vi "SEA_LOWER_LEVEL_CONTROL.vi"() -> ()   [LabVIEW 2019]
uses:
  <vilib>/rvi/Emulation/niFpgaGetClockAttributes.vi
  <vilib>/rvi/Emulation/niFpgaSctlEmulationGetInTimedLoop.vi
  <vilib>/rvi/Emulation/niFpgaEmulationReportErrorSimple.vi
  <vilib>/rvi/eio/common/nirviEmuTemplateMethod_errors.vi
  <vilib>/rvi/Emulation/niFpgaCriticalErrorInLSC.vi
  <vilib>/eio/EIONode/EIONode.xnode
  <vilib>/rvi/Arithmetic/AddSubMult/XNode/nirviSatArithmetic.xnode
panel:
  in  "Position Reset joint side":bool
  out "Position (Counts) joint side":i16
  out "Acceleration (Counts/Interval) joint side":i32
  out "Velocity (Counts/Interval) joint side":i32
  out "Loop time (position) joint side":u32
  out "Position(Radians) joint side":sgl(graph)
  in  "Position Reset":bool
  out "Position (Counts) motor side":i16
  out "Acceleration (Counts/Interval) motor side":i32
  out "Velocity (Counts/Interval) motor side":i32
  out "Loop time (position) 1 motor side":u32
  out "Position(Radians) motor side":sgl(graph)
  in  "KpGain":sgl
  in  "Tracking zero offset":sgl
  in  "reference":sgl
  out "motor direction":bool
  out "control_ip":sgl
  out "Filtered Current(M2)":sgl(graph)
  in  "Current Offset":sgl=2.4882812 format="%#_13g"
  out "Current Control Loop rate":i32
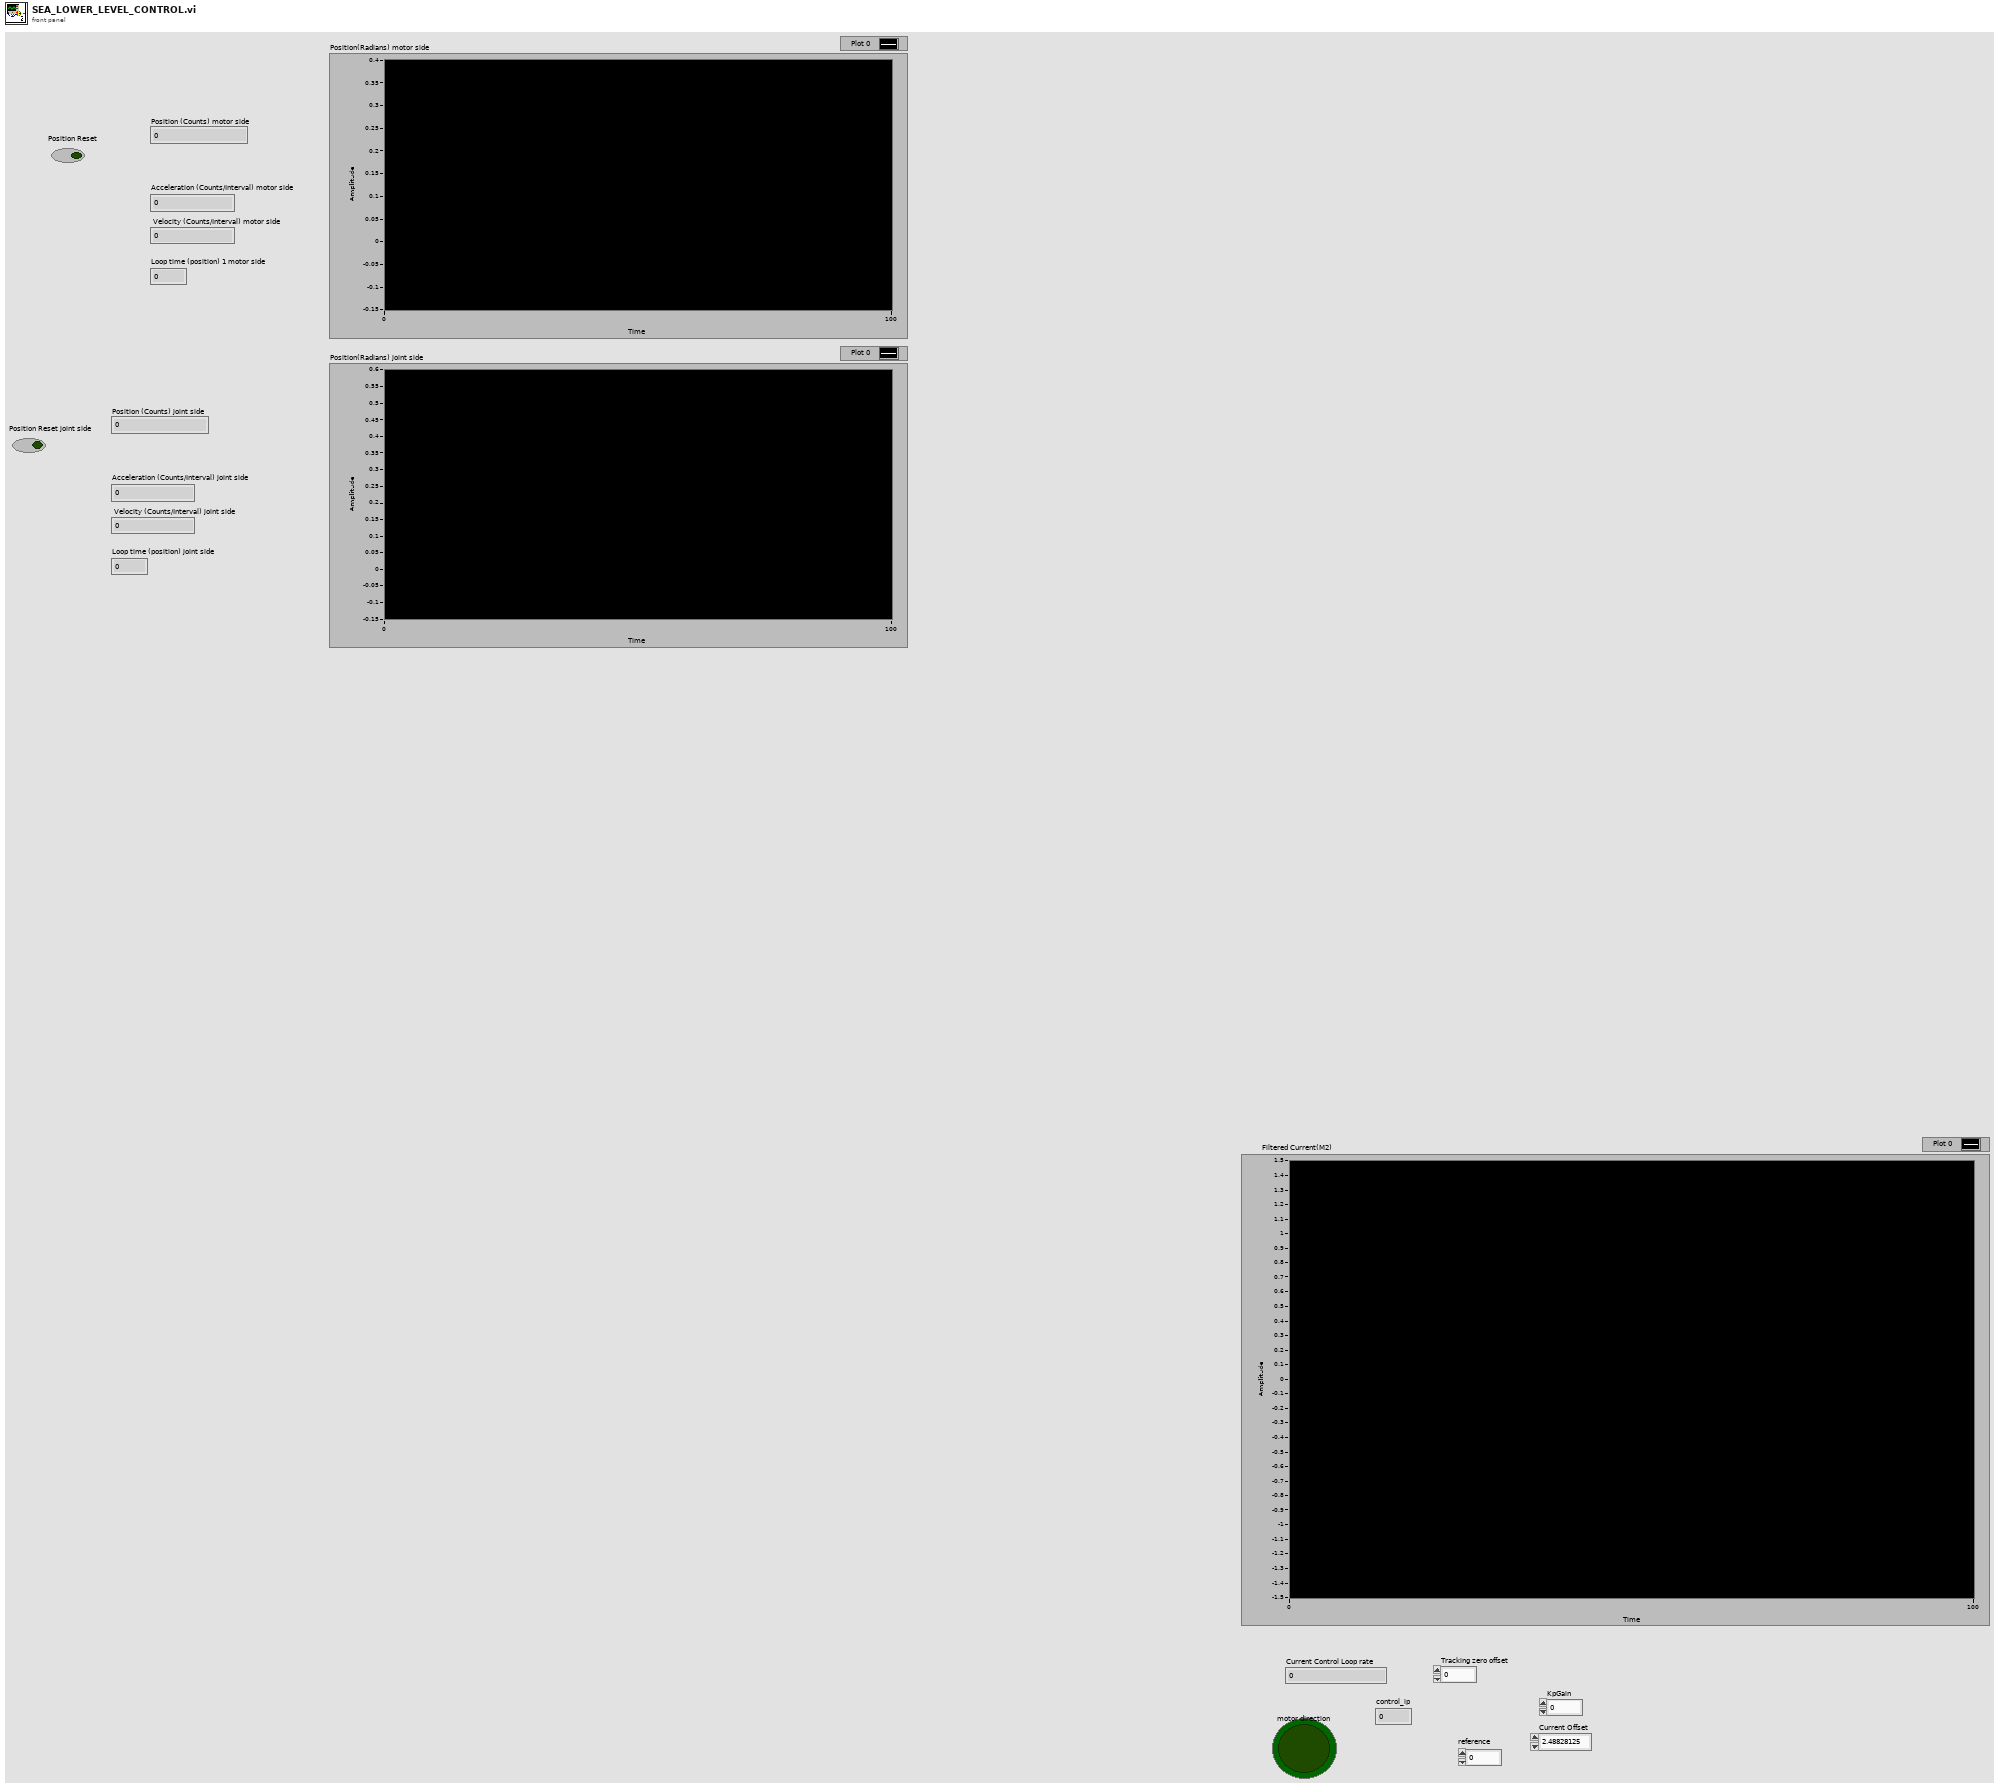
[diagram p1: front panel]
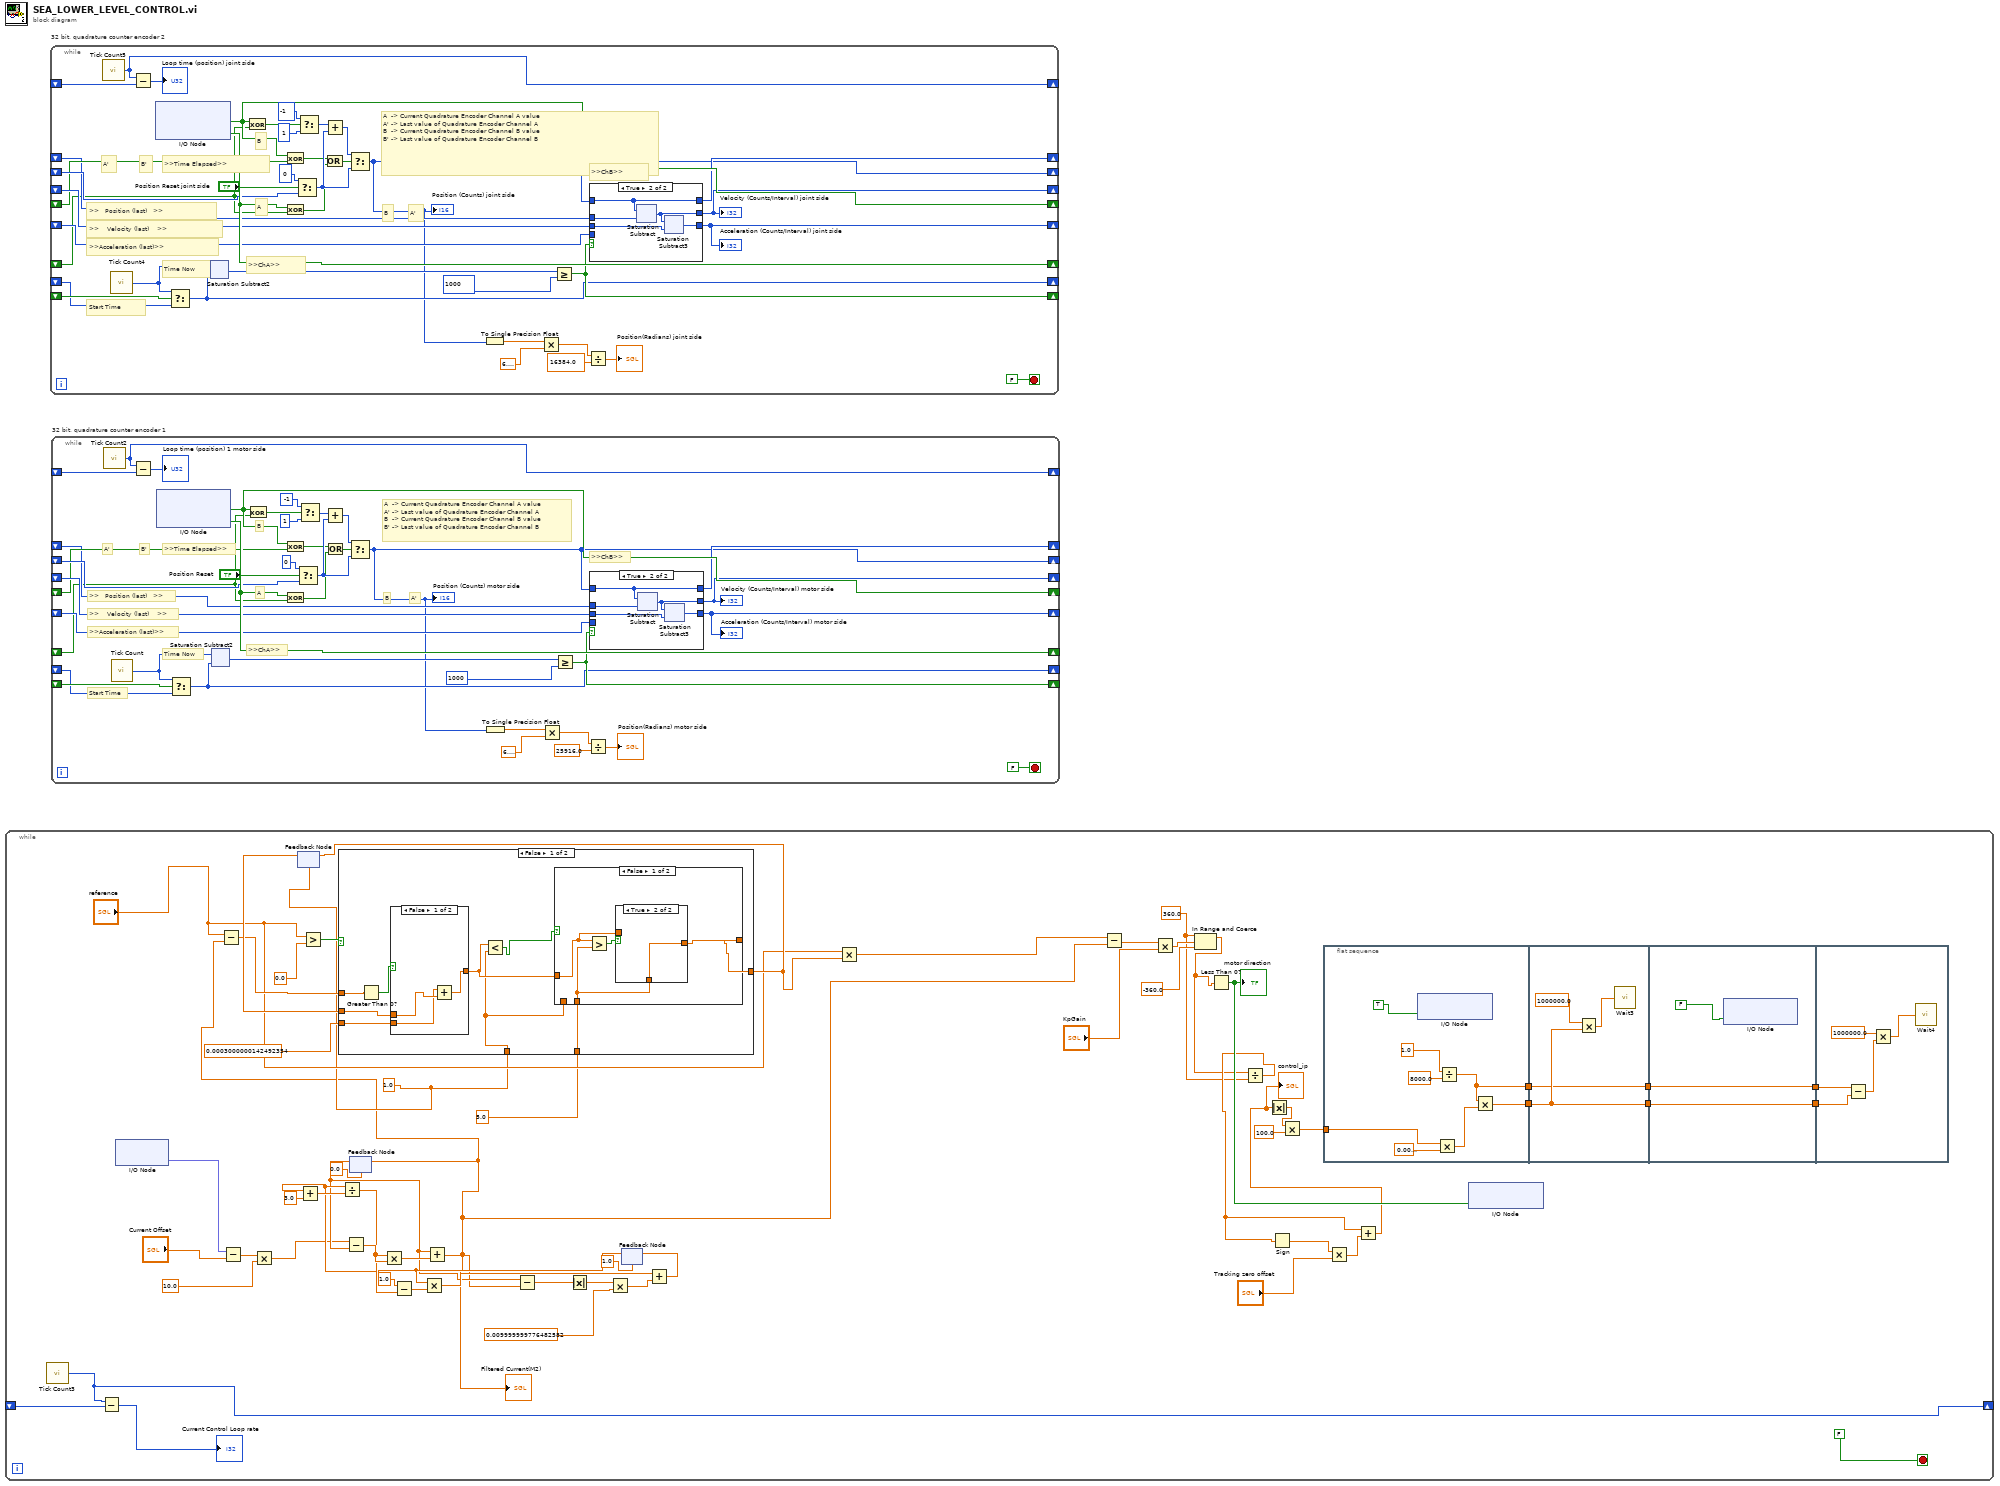
[diagram p0: block diagram]
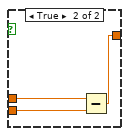
[diagram p4: hidden frame]
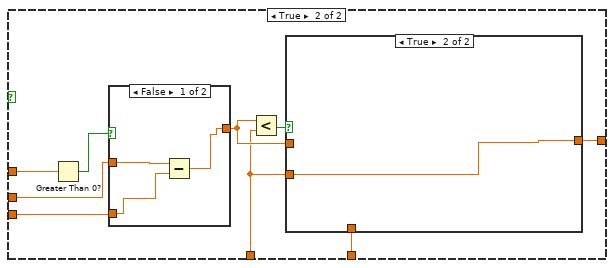
[diagram p7: hidden frame]
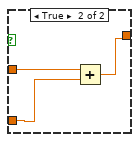
[diagram p8: hidden frame]
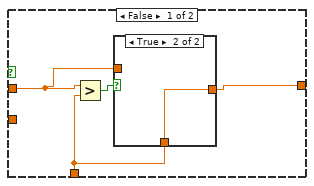
[diagram p9: hidden frame]
diagram:
  n1 = while {
    shift-right: [w22] -> _
    shift-left: _ -> [w23]
    stop <- FALSE stop-if-true
    w1 = sgl 360.0 ("upper limit")
    w11 = sgl 1.0
    n2 = call "Tick Count3"() -> ("Tick Count(uSec)"=w22:u32)
    n3 = Subtract(x=w22, y=w23) -> (x-y=→"Current Control Loop rate":u32)
    n4 = xnode "I/O Node"() -> ("AI9"=w24:fxp<+/-,24,5>)  [unwired: 1 in, 1 out]
    n5 = Subtract(x=w24, y="Current Offset") -> (x-y=w25:sgl)
    n6 = Multiply(x=w25, y=sgl 10.0) -> (x*y=w26:sgl)
    n7 = feedback #1(w11) -> (w56:sgl)
    n8 = Greater?(x="reference", y=sgl 0.0) -> (0:w57:bool)
    n9 = feedback #2(sgl 0.0) -> (w34:sgl)
    n10 = Subtract(x=w26, y=w34) -> (x-y=w42:sgl)
    n11 = feedback #3(sgl 1.0) -> (w35:sgl)
    n12 = Add(x=w35, y=sgl 3.0) -> (x+y=w44:sgl)
    n13 = Divide(x=w35, y=w44) -> (x/y=w41:sgl)
    n14 = Multiply(x=w41, y=w42) -> (x*y=w43:sgl)
    n15 = Subtract(x=sgl 1.0, y=w41) -> (x-y=w40:sgl)
    n16 = Multiply(x=w35, y=w40) -> (x*y=w39:sgl)
    n17 = Add(x=w34, y=w43) -> (x+y=w7:sgl)
    "Filtered Current(M2)" <- w7
    n18 = Subtract(x="reference", y=w7) -> (x-y=w20:sgl)
    n19 = case shown="False" w57 {
      tunnel: w20 -> [w86 w108]
      tunnel: w56 -> [w85 w106]
      tunnel: [w87 w109] -> w55
      tunnel: sgl 5.0 -> [w80 w103]
      tunnel: w11 -> [w81 w102]
      tunnel: sgl 0.0003 -> [w79 w101]
      frame False {
        n20 = Greater Than 0?(x=w86) -> (x > 0?=w84:bool)
        n21 = case shown="False" w84 {
          tunnel: w85 -> [w90 w93]
          tunnel: [w89 w92] -> w82
          tunnel: w79 -> [w88 w91]
          frame False {
            n22 = Add(x=w88, y=w90) -> (x+y=w89:sgl)
          }
          frame True {
            n23 = Subtract(x=w93, y=w91) -> (x-y=w92:sgl)
          }
        }
        n24 = Less?(x=w82, y=w81) -> (x < y?=w83:bool)
        n25 = case shown="False" w83 {
          tunnel: [w96 w100] -> w87
          tunnel: w82 -> [w95 _]
          tunnel: w81 -> [_ w100]
          tunnel: w80 -> [w94 _]
          frame False {
            n26 = Greater?(x=w95, y=w94) -> (0:w97:bool)
            n27 = case shown="True" w97 {
              tunnel: [w98 w99] -> w96
              tunnel: w95 -> [w98 _]
              tunnel: w94 -> [_ w99]
              frame False {
              }
              frame True {
              }
            }
          }
          frame True {
          }
        }
      }
      frame True {
        n28 = Greater Than 0?(x=w108) -> (x > 0?=w107:bool)
        n29 = case shown="False" w107 {
          tunnel: w106 -> [w112 w115]
          tunnel: [w111 w114] -> w104
          tunnel: w101 -> [w110 w113]
          frame False {
            n30 = Subtract(x=w112, y=w110) -> (x-y=w111:sgl)
          }
          frame True {
            n31 = Add(x=w115, y=w113) -> (x+y=w114:sgl)
          }
        }
        n32 = Less?(x=w104, y=w102) -> (x < y?=w105:bool)
        n33 = case shown="True" w105 {
          tunnel: [w118 w122] -> w109
          tunnel: w104 -> [w117 _]
          tunnel: w103 -> [w116 _]
          tunnel: w102 -> [_ w122]
          frame False {
            n34 = Greater?(x=w117, y=w116) -> (0:w119:bool)
            n35 = case shown="True" w119 {
              tunnel: [w120 w121] -> w118
              tunnel: w117 -> [w120 _]
              tunnel: w116 -> [_ w121]
              frame False {
              }
              frame True {
              }
            }
          }
          frame True {
          }
        }
      }
    }
    n36 = feedback-in #1(w55) -> ()
    n37 = feedback-in #2(w7) -> ()
    n38 = Subtract(x=w34, y=w7) -> (x-y=w38:sgl)
    n39 = Absolute Value(x=w38) -> (abs(x)=w37:sgl)
    n40 = Multiply(x=w37, y=sgl 0.01) -> (x*y=w36:sgl)
    n41 = Add(x=w39, y=w36) -> (x+y=w28:sgl)
    n42 = feedback-in #3(w28) -> ()
    n43 = Multiply(x="reference", y=w55) -> (x*y=w8:sgl)
    n44 = Subtract(x=w8, y=w7) -> (x-y=w6:sgl)
    n45 = Multiply(x=w6, y="KpGain") -> (x*y=w4:sgl)
    n46 = In Range and Coerce(upper limit=w1, x=w4, lower limit=sgl -360.0) -> (coerced(x)=w2:sgl)  [unwired: 1 out]
    n47 = Less Than 0?(x=w2) -> (x < 0?=w48:bool)
    "motor direction" <- w48
    n48 = Divide(x=w2, y=w1) -> (x/y=w13:sgl)
    n49 = Sign(1:w13) -> (0:w17:sgl)
    n50 = flat-sequence {
      tunnel: [w63] -> w54
      tunnel: [w61] -> w53
      tunnel: w45 -> [w59]
      tunnel: w54 -> [w68]
      tunnel: [w68] -> w52
      tunnel: w53 -> [w67]
      tunnel: [w67] -> w51
      tunnel: w52 -> [w73]
      tunnel: [w73] -> w50
      tunnel: w51 -> [w72]
      tunnel: [w72] -> w49
      tunnel: w50 -> [w78]
      tunnel: w49 -> [w74]
      frame #0 {
        n51 = xnode "I/O Node"("RMC/DIO33"=TRUE) -> ()  [unwired: 1 in, 1 out]
        n52 = Multiply(x=w59, y=sgl 0.01) -> (x*y=w64:sgl)
        n53 = Divide(x=sgl 1.0, y=sgl 8000.0) -> (x/y=w61:sgl)
        n54 = Multiply(x=w61, y=w64) -> (x*y=w63:sgl)
      }
      frame #1 {
        n55 = Multiply(x=sgl 1000000.0, y=w68) -> (x*y=w70:sgl)
        n56 = call "Wait3"("Count(uSec)"=w70) -> ()  [unwired: 1 out]
      }
      frame #2 {
        n57 = xnode "I/O Node"("RMC/DIO33"=FALSE) -> ()  [unwired: 1 in, 1 out]
      }
      frame #3 {
        n58 = Subtract(x=w74, y=w78) -> (x-y=w77:sgl)
        n59 = Multiply(x=sgl 1000000.0, y=w77) -> (x*y=w76:sgl)
        n60 = call "Wait4"("Count(uSec)"=w76) -> ()  [unwired: 1 out]
      }
    }
    n61 = Multiply(x=w17, y="Tracking zero offset") -> (x*y=w15:sgl)
    n62 = Add(x=w13, y=w15) -> (x+y=w14:sgl)
    "control_ip" <- w14
    n63 = Absolute Value(x=w14) -> (abs(x)=w47:sgl)
    n64 = Multiply(x=w47, y=sgl 100.0) -> (x*y=w45:sgl)
    n65 = xnode "I/O Node"("RMC/DIO34"=w48) -> ()  [unwired: 1 in, 1 out]
  }
  n66 = while "32 bit, quadrature counter encoder 2" {
    shift-right: [w151] -> _
    shift-left: _ -> [w139]
    shift-right: [w130] -> _
    shift-left: _ -> [w148]
    shift-right: [w150] -> _
    shift-left: _ -> [w131]
    shift-right: [w145] -> _
    shift-left: _ -> [w147]
    shift-right: [w141] -> _
    shift-left: _ -> [w146]
    shift-right: [w136] -> _
    shift-left: _ -> [w135]
    shift-right: [w137] -> _
    shift-left: _ -> [w143]
    shift-right: [w138] -> _
    shift-left: _ -> [w140]
    shift-right: [w132] -> _
    shift-left: _ -> [w134]
    stop <- FALSE stop-if-true
    # "A  -> Current Quadrature Encoder Channel A value\nA' -> Last value of Quadrature Encoder Channel A\nB  -> Current Quadrature Encoder Channel B value\nB' -> Last value of Quadrature Encoder Channel B"
    # ">>Acceleration (last)>>"
    # "Start Time"
    # "A'"
    # "B"
    # "A'"
    # "A"
    # "B'"
    # "B"
    # ">>ChB>>"
    # ">>ChA>>"
    # ">>    Velocity (last)    >>"
    # ">>   Position (last)   >>"
    # "Time Now"
    # ">>Time Elapsed>>"
    n67 = call "Tick Count5"() -> ("Tick Count(Ticks)"=w132:u32)
    n68 = call "Tick Count4"() -> ("Tick Count(uSec)"=w142:u32)
    n69 = Subtract(x=w132, y=w134) -> (x-y=→"Loop time (position) joint side":u32)
    n70 = xnode "I/O Node"() -> ("RMC/DIO44"=w151:bool, "RMC/DIO42"=w150:bool)  [unwired: 2 in, 2 out]
    n71 = Select(t=w142, s=w147, f=w146) -> (s? t:f=w141:u32)
    n72 = xnode ("Saturation Subtract2")("x"=w142, "y"=w141) -> ("x-y"=w144:u32)
    n73 = Exclusive Or(1:w131, 2:w151) -> (0:w152:bool)
    n74 = Exclusive Or(1:w139, 2:w151) -> (0:w153:bool)
    n75 = Exclusive Or(1:w131, 2:w150) -> (0:w154:bool)
    n76 = Select(t=0 ("32 bit"), s="Position Reset joint side", f=w148) -> (s? t:f=w159:i32)
    n77 = Select(t=-1 ("32 bit"), s=w152, f=1 ("32 bit")) -> (s? t:f=w157:i32)
    n78 = Add(x=w157, y=w159) -> (x+y=w161:i32)
    n79 = Or(x=w153, y=w154) -> (x .or. y?=w149:bool)
    n80 = Select(t=w161, s=w149, f=w159) -> (s? t:f=w130:i32)
    "Position (Counts) joint side" <- w130
    n81 = To Single Precision Float(number=w130) -> (single precision float=w129:sgl)
    n82 = Multiply(x=w129, y=sgl 6.2831855) -> (x*y=w127:sgl)
    n83 = Greater Or Equal?(x=w144, y=u32 1000) -> (x >= y?=w145:bool)
    n84 = Divide(x=w127, y=sgl 16384.0) -> (x/y=→"Position(Radians) joint side":sgl)
    n85 = case shown="True" w145 {
      tunnel: w130 -> [_ w175]
      tunnel: w135 -> [w172 w179]
      tunnel: [w174 w178] -> w137
      tunnel: w143 -> [w174 w177]
      tunnel: [w173 w176] -> w138
      tunnel: w140 -> [w173 _]
      tunnel: [w172 w175] -> w136
      frame False {
      }
      frame True {
        n86 = xnode ("Saturation Subtract")("x"=w175, "y"=w179) -> ("x-y"=w178:i32)
        n87 = xnode ("Saturation Subtract3")("x"=w178, "y"=w177) -> ("x-y"=w176:i32)
      }
    }
    "Acceleration (Counts/Interval) joint side" <- w138
    "Velocity (Counts/Interval) joint side" <- w137
  }
  n88 = while "32 bit, quadrature counter encoder 1" {
    shift-right: [w244] -> _
    shift-left: _ -> [w232]
    shift-right: [w223] -> _
    shift-left: _ -> [w241]
    shift-right: [w243] -> _
    shift-left: _ -> [w224]
    shift-right: [w238] -> _
    shift-left: _ -> [w240]
    shift-right: [w234] -> _
    shift-left: _ -> [w239]
    shift-right: [w229] -> _
    shift-left: _ -> [w228]
    shift-right: [w230] -> _
    shift-left: _ -> [w236]
    shift-right: [w231] -> _
    shift-left: _ -> [w233]
    shift-right: [w225] -> _
    shift-left: _ -> [w227]
    stop <- FALSE stop-if-true
    # "A  -> Current Quadrature Encoder Channel A value\nA' -> Last value of Quadrature Encoder Channel A\nB  -> Current Quadrature Encoder Channel B value\nB' -> Last value of Quadrature Encoder Channel B"
    # ">>Acceleration (last)>>"
    # "Start Time"
    # "A'"
    # "B"
    # "A'"
    # "A"
    # "B'"
    # "B"
    # ">>ChB>>"
    # ">>ChA>>"
    # ">>    Velocity (last)    >>"
    # ">>   Position (last)   >>"
    # "Time Now"
    # ">>Time Elapsed>>"
    n89 = call "Tick Count2"() -> ("Tick Count(Ticks)"=w225:u32)
    n90 = call "Tick Count"() -> ("Tick Count(uSec)"=w235:u32)
    n91 = Subtract(x=w225, y=w227) -> (x-y=→"Loop time (position) 1 motor side":u32)
    n92 = xnode "I/O Node"() -> ("RMC/DIO10"=w244:bool, "RMC/DIO9"=w243:bool)  [unwired: 2 in, 2 out]
    n93 = Select(t=w235, s=w240, f=w239) -> (s? t:f=w234:u32)
    n94 = xnode ("Saturation Subtract2")("x"=w235, "y"=w234) -> ("x-y"=w237:u32)
    n95 = Exclusive Or(1:w224, 2:w244) -> (0:w245:bool)
    n96 = Exclusive Or(1:w232, 2:w244) -> (0:w246:bool)
    n97 = Exclusive Or(1:w224, 2:w243) -> (0:w247:bool)
    n98 = Select(t=0 ("32 bit"), s="Position Reset", f=w241) -> (s? t:f=w252:i32)
    n99 = Select(t=-1 ("32 bit"), s=w245, f=1 ("32 bit")) -> (s? t:f=w250:i32)
    n100 = Add(x=w250, y=w252) -> (x+y=w254:i32)
    n101 = Or(x=w246, y=w247) -> (x .or. y?=w242:bool)
    n102 = Select(t=w254, s=w242, f=w252) -> (s? t:f=w223:i32)
    "Position (Counts) motor side" <- w223
    n103 = To Single Precision Float(number=w223) -> (single precision float=w222:sgl)
    n104 = Multiply(x=w222, y=sgl 6.2831855) -> (x*y=w220:sgl)
    n105 = Greater Or Equal?(x=w237, y=u32 1000) -> (x >= y?=w238:bool)
    n106 = Divide(x=w220, y=sgl 25916.0) -> (x/y=→"Position(Radians) motor side":sgl)
    n107 = case shown="True" w238 {
      tunnel: w223 -> [_ w268]
      tunnel: w228 -> [w265 w272]
      tunnel: [w267 w271] -> w230
      tunnel: w236 -> [w267 w270]
      tunnel: [w266 w269] -> w231
      tunnel: w233 -> [w266 _]
      tunnel: [w265 w268] -> w229
      frame False {
      }
      frame True {
        n108 = xnode ("Saturation Subtract")("x"=w268, "y"=w272) -> ("x-y"=w271:i32)
        n109 = xnode ("Saturation Subtract3")("x"=w271, "y"=w270) -> ("x-y"=w269:i32)
      }
    }
    "Acceleration (Counts/Interval) motor side" <- w231
    "Velocity (Counts/Interval) motor side" <- w230
  }
